vi "shim_heater_set_state.vi"(8 "error in":errorcluster, 9 "state_ch2":bool, 10 "state_ch1":bool, 11 "conn_id_in":refnum<k5>) -> (0 "error out":errorcluster, 1 "ch2":bool, 2 "ch1":bool, 3 "conn_id_out":refnum<k5>, 4 "status":bool, 6 "message":string)   [LabVIEW 2019]
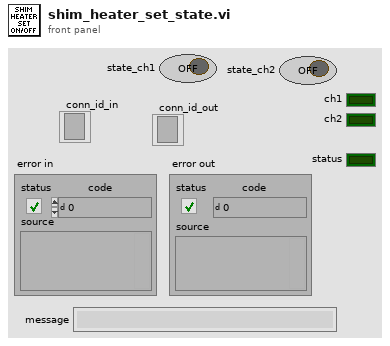
[diagram p1: front panel]
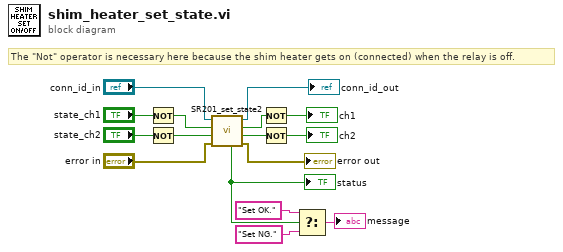
[diagram p0: block diagram]
diagram:
  # "The \"Not\" operator is necessary here because the shim heater gets on (connected) when the relay is off."
  n1 = Not(x="state_ch1") -> (.not. x?=w12:bool)
  n2 = Not(x="state_ch2") -> (.not. x?=w11:bool)
  n3 = call "SR201_set_state2.vi"("error in"="error in", "state_ch2"=w11, "state_ch1"=w12, "conn_id_in"="conn_id_in") -> ("error out"=→"error out":errorcluster, "ch2"=w6:bool, "ch1"=w5:bool, "conn_id_out"=→"conn_id_out":refnum<k5>, "status"=w1:bool)  [unwired: 2 in, 1 out]
  "status" <- w1
  n4 = Not(x=w5) -> (.not. x?=→"ch1":bool)
  n5 = Not(x=w6) -> (.not. x?=→"ch2":bool)
  n6 = Select(t="Set OK." ("message"), s=w1, f="Set NG." ("message")) -> (s? t:f=→"message":string)
